vi "State and Done.vi"(11 "Async Authorization in":refnum<class "Async Authorization.lvclass">) -> (1 "Done?":bool, 2 "State":T1)   [LabVIEW 2020, in "OAuth2.lvlib" / "Async Authorization.lvclass"]
doc: "Returns the current state of the Authorization flow and whether it has completed or not.\n\n<b>Initialize</b> - The auth flow is being configured.\n<b>Request</b> - The user is being directed to the authorization portal in a browser.\n<b>WaitAuth</b> - The authorization is waiting on the user to grant the authorization.\n<b>GetToken</b> - The user has provided authorization and the token is being requested.\n<b>RefreshToken</b> - A renewed token is being retrieved with the refresh token.\n<b>Complete</b> - The authorization has succeeded and is ready for use.\n<b>Failed</b> - The authorization failed. This could be due to improper configuration, the user cancelling the authorization, or the user not responding within the timeout."
uses:
  Async Authorization.lvclass
  Async Auth State.ctl
  OAuth2.lvlib
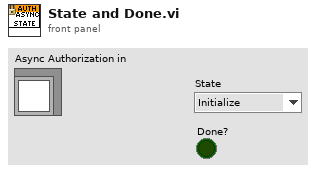
[diagram p1: front panel]
types:
  T1 = typedef "OAuth2.lvlib/Async Auth State.ctl" = enum16{"Initialize", "Request", "WaitAuth", "GetToken", "RefreshToken", "Complete", "Failed"}
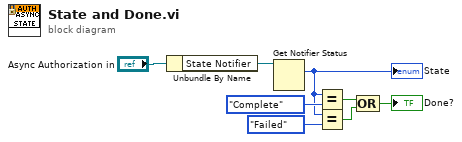
[diagram p0: block diagram]
diagram:
  n1 = Unbundle By Name("Async Authorization in") -> ("State Notifier"=w7:refnum<notifier>)
  n2 = Get Notifier Status(notifier=w7) -> (current notification=w4:T1)  [unwired: 1 in, 4 out]
  "State" <- w4
  n3 = Equal?(x=w4, y=Async_Auth_State."Complete") -> (x = y?=w3:bool)
  n4 = Equal?(x=w4, y=Async_Auth_State."Failed") -> (x = y?=w2:bool)
  n5 = Compound Arithmetic op=OR(w3, w2) -> (→"Done?":bool)
